vi "Vision Processing.vi"(4 "error in (no error)":errorcluster, 7 "Image Size":T3=enum."320x240") -> (2 "Target Y":dbl, 3 "Target  X":dbl)   [LabVIEW 2015]
uses:
  <vilib>/Rock Robotics/WPI/Camera/WPI_CameraImageSize.ctl
  <vilib>/Rock Robotics/WPI/Camera/WPI_CameraWhite Balance Values.ctl
  <vilib>/Rock Robotics/WPI/Camera/WPI_CameraExposure Values.ctl
  <vilib>/Rock Robotics/WPI/Camera/WPI_CameraFrameRate.ctl
  Vision Support Code/Camera Types.ctl
  Robot Global Data.vi
  <vilib>/vision/NI_Vision_Development_Module.lvlib
panel:
  out "Highest Avg Score":dbl
  in  "Min Score Threshold":i32=75
  out "Detected Targets":T1(array[cluster]) {"Normalized Rect"."Numeric 5" format="%#_2g"; "Normalized Rect"."Numeric 3" format="%#_2g"; "Normalized Rect"."Numeric 2" format="%#_2g"; "Normalized Rect"."Numeric" format="%#_2g"}
  out "Sorted Particle Scores":T2(array[cluster]) {"Moment Factor" format="%#_3g"; "Aspect Ratio" format="%#_3g"; "Area to CH" format="%#_3g"; "X" format="%#_3g"; "Y" format="%#_3g"}
  in  "Display Original":bool=TRUE
  in  "Display Mask":bool=TRUE
  out "fps":dbl
  in  "Emphasize Limit Tests":bool=TRUE
  in  "Aspect Fudge Factor":dbl=1.0
  in  "Score Threshold":dbl=75.0
  out "ms to process":u32
  out "Qualified Particles":i32
  in  "LED Color":T4={"Hue"={111.0, 149.0}, "Sat"={35.0, 255.0}, "Val"={93.0, 255.0}} {"Hue" scale=0.0..255.0 scale format="%#_3g"}
  out "Masked":T5(plugin-control)
  out "Original Image":T5(plugin-control)
  # "NOTE:\nFor best results, lower the camera\nexposure."
  # "This is only the initial camera size.\nOther camera setup is done\non the diagram. Notice it is set\nonce before the loop but can be\nupdated within the loop if needed."
  # "Instructions:\nUse LED Color to threshold and build particles. Adjust calibration if needed.\nDisplays are very useful for debugging, but will slow down execution, so you\nmay want to disable once working.\nAnnotations show the rectangle and the scores from top to bottom.\nChange camera setting on diagram."
  # "x"
  # "y"
  # "Density Profile"
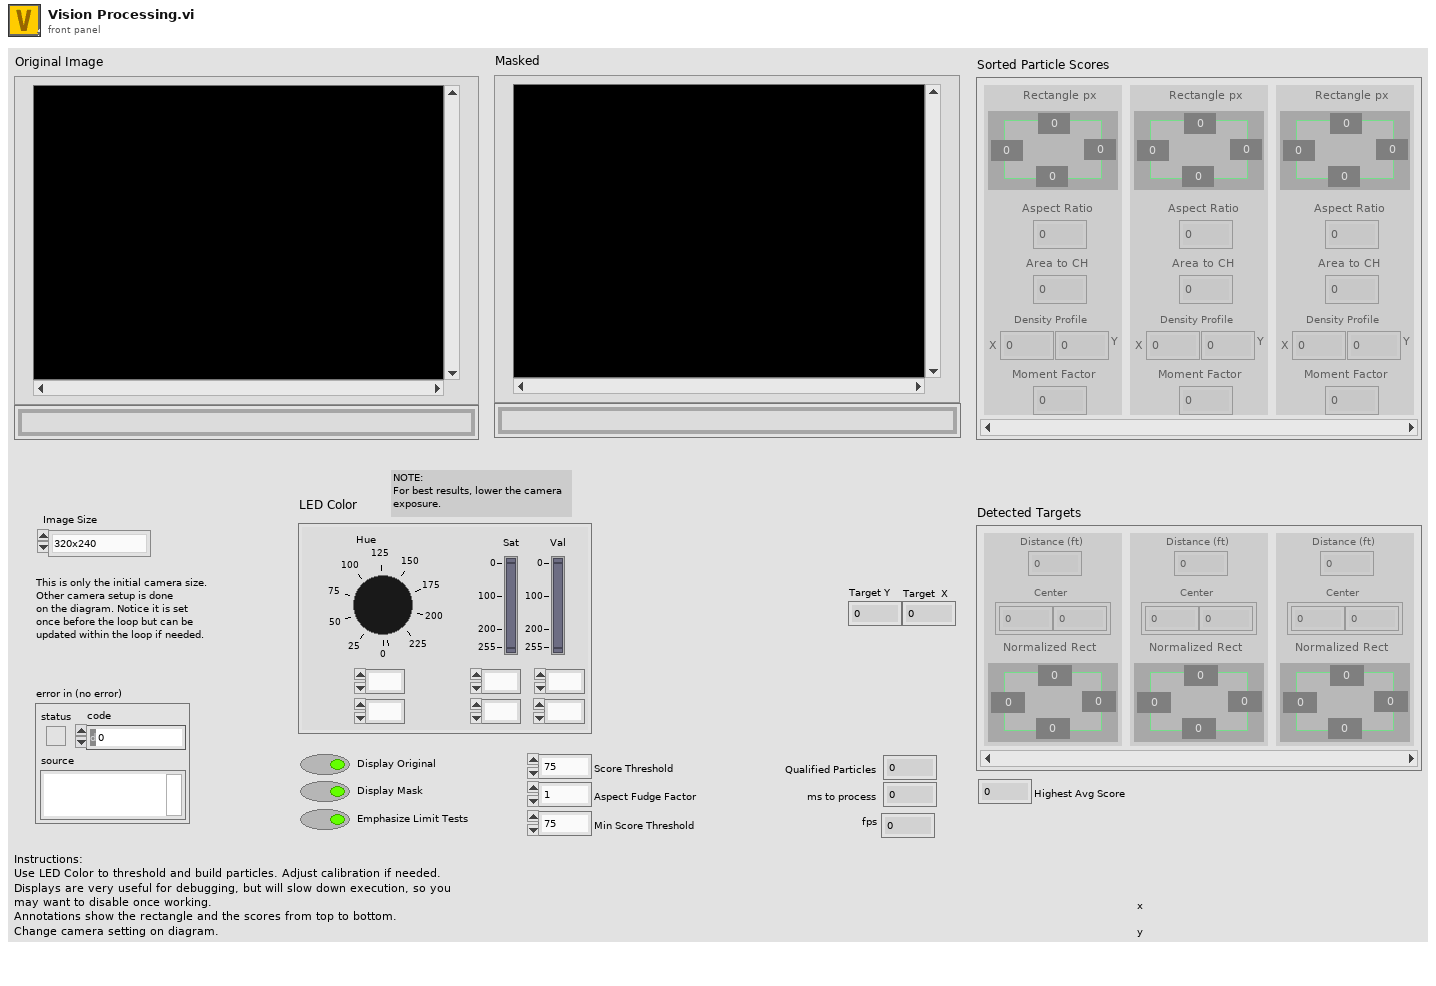
[diagram p1: front panel]
types:
  T1 = cluster{"Distance (ft)":dbl, "Center":cluster{dbl, dbl}, "Normalized Rect":cluster{"Numeric":dbl, "Numeric 2":dbl, "Numeric 3":dbl, "Numeric 5":dbl}}[]
  T2 = cluster{"Rectangle px":cluster{"Numeric":dbl, "Numeric 2":dbl, "Numeric 3":dbl, "Numeric 5":dbl}, "Aspect Ratio":dbl, "Area to CH":dbl, "X":dbl, "Y":dbl, "Moment Factor":dbl}[]
  T3 = typedef "WPI_CameraImageSize.ctl" = enum16{"640x480", "320x240", "160x120", "Custom"}
  T4 = cluster{"Hue":cluster{dbl, dbl}, "Sat":cluster{dbl, dbl}, "Val":cluster{dbl, dbl}}
  T5 = typedef "IMAQ Image.ctl" = refnum<image>
  T6 = typedef "WPI_CameraFrameRate.ctl" = u32
  T7 = typedef "WPI_CameraExposure Values.ctl" = enum16{"Auto", "Flicker-free 50 Hz", "Flicker-free 60 Hz", "Hold current", "Custom"}
  T8 = typedef "WPI_CameraWhite Balance Values.ctl" = enum16{"Auto", "Fixed indoor", "Fixed outdoor 1", "Fixed outdoor 2", "Fixed fluorescent 1", "Fixed fluorescent 2", "Hold current", "Custom"}
  T9 = typedef "Particle Parameters" = i32
  T10 = typedef "Image Type" = u32
  T11 = typedef "WPI_CameraDevRef.ctl" = cluster{"Camera Address":string, "CameraStatus":errorcluster}
  T12 = typedef "Camera Types.ctl" = enum16{"206", "1011", "1013", "MS HD3000 square", "MS HD3000 640x480"}
  T13 = cluster{"Bounding box":cluster{"left":dbl, "top":dbl, "right":dbl, "bottom":dbl}, "Aspect Ratio":dbl, "Area to CH":dbl, "X Mask":dbl, "Y Mask":dbl, "Moment":dbl}[]
  T14 = cluster{"Rectangle":cluster{"Numeric":dbl, "Numeric 2":dbl, "Numeric 3":dbl, "Numeric 5":dbl}, "L":dbl, "Area to CH":dbl, "X":dbl, "Y":dbl, "Moment Factor":dbl}[]
  T15 = cluster{"Distance (ft)":dbl, "Center":cluster{dbl, dbl}, "Normalized Rect":cluster{"Numeric":dbl, "Numeric 2":dbl, "Numeric 3":dbl, "Numeric 5":dbl}}
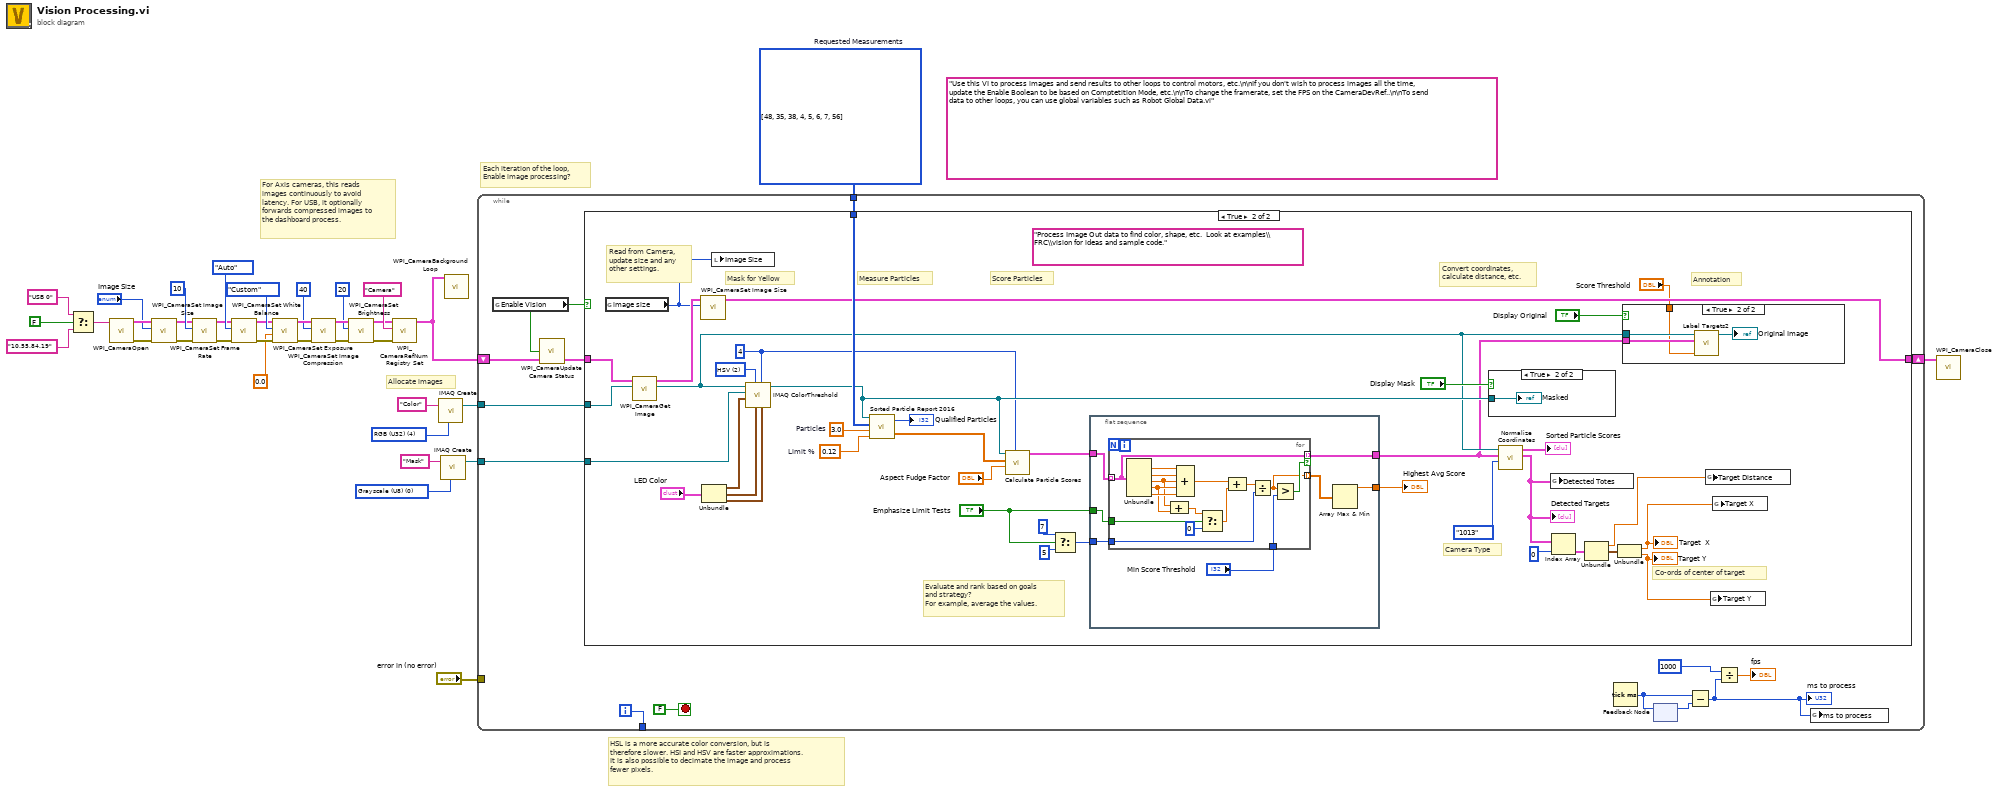
[diagram p0: block diagram]
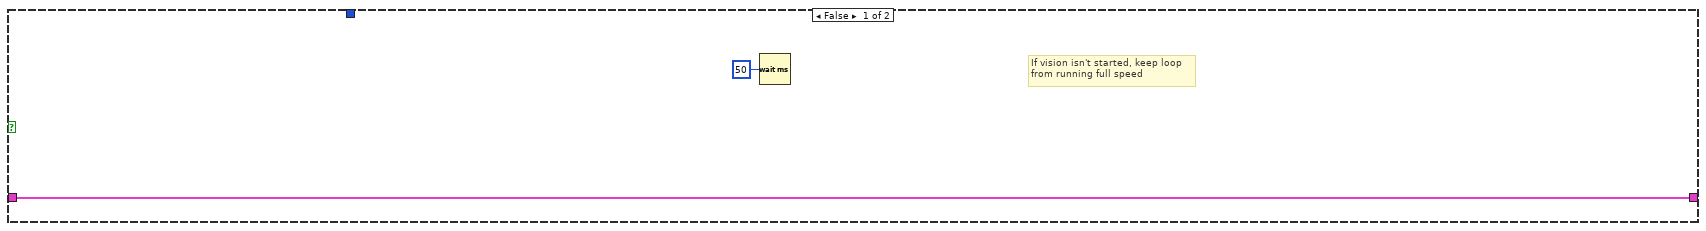
[diagram p2: hidden frame]
diagram:
  (unwired) "Use this VI to process images and send results to other loops to control motors, etc.\n\nIf you don't wish to process images all the time, update the Enable Boolean to be based on Comptetition Mode, etc.\n\nTo change the framerate, set the FPS on the CameraDevRef..\n\nTo send data to other loops, you can use global variables such as Robot Global Data.vi"
  w30 = T9[] [48, 35, 38, 4, 5, 6, 7, 56] items=["Center of Mass X", "Center of Mass Y", "First Pixel X", "First Pixel Y", "Bounding Rect Left", "Bounding Rect Top", "Bounding Rect Right", "Bounding Rect Bottom", "Max Feret Diameter Start X", "Max Feret Diameter Start Y", "Max Feret Diameter End X", "Max Feret Diameter End Y", "Max Horiz. Segment Length Left", "Max Horiz. Segment Length Right", "Max Horiz. Segment Length Row", "-", "Bounding Rect Width", "Bounding Rect Height", "Bounding Rect Diagonal", "Perimeter", "Convex Hull Perimeter", "Holes' Perimeter", "Max Feret Diameter", "Equivalent Ellipse Major Axis", "Equivalent Ellipse Minor Axis", "Equivalent Ellipse Minor Axis (Feret)", "Equivalent Rect Long Side", "Equivalent Rect Short Side", "Equivalent Rect Diagonal", "Equivalent Rect Short Side (Feret)", "Average Horiz. Segment Length", "Average Vert. Segment Length", "Hydraulic Radius", "Waddel Disk Diameter", "-", "Area", "Holes' Area", "Particle & Holes' Area", "Convex Hull Area", "Image Area", "-", "Number of Holes", "Number of Horiz. Segments", "Number of Vert. Segments", "-", "Orientation", "Max Feret Diameter Orientation", "-", "% Area/Image Area", "% Area/(Particle & Holes' Area)", "Ratio of Equivalent Ellipse Axes", "Ratio of Equivalent Rect Sides", "-", "Elongation Factor", "Compactness Factor", "Heywood Circularity Factor", "Type Factor", "-", "Sum X", "Sum Y", "Sum XX", "Sum XY", "Sum YY", "Sum XXX", "Sum XXY", "Sum XYY", "Sum YYY", "-", "Moment of Inertia XX", "Moment of Inertia XY", "Moment of Inertia YY", "Moment of Inertia XXX", "Moment of Inertia XXY", "Moment of Inertia XYY", "Moment of Inertia YYY", "Norm. Moment of Inertia XX", "Norm. Moment of Inertia XY", "Norm. Moment of Inertia YY", "Norm. Moment of Inertia XXX", "Norm. Moment of Inertia XXY", "Norm. Moment of Inertia XYY", "Norm. Moment of Inertia YYY", "Hu Moment 1", "Hu Moment 2", "Hu Moment 3", "Hu Moment 4", "Hu Moment 5", "Hu Moment 6", "Hu Moment 7"]  # Requested Measurements
  w33 = T10 0 items=["Grayscale (U8)", "Grayscale (I16)", "Grayscale (SGL)", "Complex (CSG)", "RGB (U32)", "HSL (U32)", "RGB (U64)", "Grayscale (U16)"] ("Image Type")
  w35 = T10 4 items=["Grayscale (U8)", "Grayscale (I16)", "Grayscale (SGL)", "Complex (CSG)", "RGB (U32)", "HSL (U32)", "RGB (U64)", "Grayscale (U16)"] ("Image Type")
  # "Each iteration of the loop,\nEnable image processing?"
  # "HSL is a more accurate color conversion, but is\ntherefore slower. HSI and HSV are faster approximations.\nIt is also possible to decimate the image and process\nfewer pixels."
  # "For Axis cameras, this reads\nimages continuously to avoid\nlatency. For USB, it optionally\nforwards compressed images to\nthe dashboard process."
  # "Allocate images"
  n1 = Select(t="USB 0" ("format string"), s=FALSE ("dot notation? (F)"), f="10.55.84.19" ("format string")) -> (s? t:f=w29:string)
  n2 = call <vilib>:"WPI_CameraOpen.vi"("Camera Address"=w29) -> ("error out"=w17:errorcluster, "CameraDevRef"=w16:T11)  [unwired: 1 in, 8 out]
  n3 = call <vilib>:"WPI_CameraSet Image Size.vi"("error in (no error)"=w17, "Image Size"="Image Size", "CameraDevRef"=w16) -> ("error out"=w18:errorcluster, "CameraDevRef Out"=w15:T11)  [unwired: 1 in, 6 out]
  n4 = call <vilib>:"WPI_CameraSet Frame Rate.vi"("error in (no error)"=w18, "Frame Rate (fps)"=T6 10, "CameraDevRef"=w15) -> ("error out"=w19:errorcluster, "CameraDevRef Out"=w13:T11)  [unwired: 7 out]
  n5 = call <vilib>:"WPI_CameraSet White Balance.vi"("error in (no error)"=w19, "White Balance"=WPI_CameraWhite_Balance_Values."Auto", "CameraDevRef"=w13) -> ("error out"=w20:errorcluster, "CameraDevRef Out"=w14:T11)  [unwired: 1 in, 6 out]
  n6 = call <vilib>:"WPI_CameraSet Exposure.vi"("error in (no error)"=w20, "Exposure (%)"=0.0, "Exposure"=WPI_CameraExposure_Values."Custom", "CameraDevRef"=w14) -> ("error out"=w21:errorcluster, "CameraDevRef Out"=w11:T11)  [unwired: 6 out]
  n7 = call <vilib>:"WPI_CameraSet Image Compression.vi"("error in (no error)"=w21, "Compression"=40, "CameraDevRef"=w11) -> ("error out"=w22:errorcluster, "CameraDevRef Out"=w12:T11)  [unwired: 7 out]
  n8 = call <vilib>:"WPI_CameraSet Brightness.vi"("error in (no error)"=w22, "Brightness"=20, "CameraDevRef"=w12) -> ("error out"=w23:errorcluster, "CameraDevRef Out"=w2:T11)  [unwired: 7 out]
  n9 = call <vilib>:"WPI_CameraRefNum Registry Set.vi"("error in (no error)"=w23, "refnum name"="Camera", "CameraDevRef"=w2) -> ("CameraDevRef"=w7:T11)  [unwired: 1 in, 7 out]
  n10 = call "IMAQ Create"("Image Name"="Color", "Image Type"=w35) -> ("New Image"=w34:T5)  [unwired: 2 in, 2 out]
  n11 = call "IMAQ Create"("Image Name"="Mask", "Image Type"=w33) -> ("New Image"=w31:T5)  [unwired: 2 in, 2 out]
  n12 = call <vilib>:"WPI_CameraBackground Loop.vi"("CameraDevRef"=w7) -> ()  [unwired: 11 in]
  n13 = while {
    tunnel: w34 -> [w45]
    tunnel: w31 -> [w49]
    tunnel: w30 -> [w48]
    tunnel: "error in (no error)" -> [_]
    tunnel: [w44] -> _
    shift-right: [w40] -> w3
    shift-left: w7 -> [w42]
    i -> [w44]
    stop <- FALSE stop-if-true
    n14 = global read "Robot Global Data.vi" "Enable Vision"() -> (w43:bool)
    n15 = call <vilib>:"WPI_CameraUpdate Camera Status.vi"("CameraDevRef In"=w42, "Enable Vision"=w43) -> ("CameraDevRef Out"=w41:T11)  [unwired: 3 in]
    n16 = case shown="True" w43 {
      tunnel: w49 -> [_ w91]
      tunnel: w48 -> [_ w86]
      tunnel: w41 -> [w51 w82]
      tunnel: w45 -> [_ w81]
      tunnel: [w51 w79] -> w40
      frame False {
        # "If vision isn't started, keep loop\nfrom running full speed"
        n17 = Wait (ms)(milliseconds to wait=u32 50) -> ()  [unwired: 1 out]
      }
      frame True {
        w63 = 4 ("Replace Value")
        w76 = u16 2 items=["RGB", "HSL", "HSV", "HSI"] ("Color Mode")
        (unwired) "Process Image Out data to find color, shape, etc.  Look at examples\\FRC\\vision for ideas and sample code."
        w83 = 0.12  # Limit %
        w85 = 3.0  # Particles
        # "Co-ords of center of target"
        # "Camera Type"
        # "Evaluate and rank based on goals\nand strategy?\nFor example, average the values."
        # "Read from Camera,\nupdate size and any\nother settings."
        # "Measure Particles"
        # "Convert coordinates,\ncalculate distance, etc."
        # "Annotation"
        # "Score Particles"
        # "Mask for Yellow"
        n18 = global read "Robot Global Data.vi" "image size"() -> (w62:T3)
        n19 = call <vilib>:"WPI_CameraGet Image.vi"("Image"=w81, "CameraDevRef"=w82) -> ("Image Out"=w66:T5, "CameraDevRef Out"=w80:T11)  [unwired: 7 in, 1 out]
        n20 = call <vilib>:"WPI_CameraSet Image Size.vi"("Image Size"=w62, "CameraDevRef"=w80) -> ("CameraDevRef Out"=w79:T11)  [unwired: 2 in, 7 out]
        n21 = Unbundle("LED Color") -> ("Hue"=w90:cluster{dbl, dbl}, "Sat"=w89:cluster{dbl, dbl}, "Val"=w88:cluster{dbl, dbl})
        n22 = local write "Image Size"(w62) -> ()
        n23 = call "IMAQ ColorThreshold"("Blue or Luma or Val or Inten Range"=w88, "Replace Value"=w63, "Green or Sat Range"=w89, "Color Mode"=w76, "Red or Hue Range"=w90, "Image Dst"=w91, "Image Src"=w66) -> ("Image Dst Out"=w75:T5)  [unwired: 3 in, 1 out]
        n24 = call "Sorted Particle Report 2016.vi"("Min Area Size %"=w83, "Particle Count Limit"=w85, "Pixel Measurements"=w86, "Image in"=w75) -> ("Sorted Data"=w74:dbl[][], "Particles"=→"Qualified Particles":i32)
        n25 = call "Calculate Particle Scores.vi"("Pixel Value"=w63, "Aspect Fudge Factor"="Aspect Fudge Factor", "Sorted Data"=w74, "Image in"=w75) -> ("Scores"=w72:T13)  [unwired: 7 in]
        n26 = Select(t=7, s="Emphasize Limit Tests", f=5) -> (s? t:f=w69:i32)
        n27 = flat-sequence {
          tunnel: w72 -> [w102]
          tunnel: w69 -> [w100]
          tunnel: [w103] -> w68
          tunnel: [w97] -> w65
          tunnel: "Emphasize Limit Tests" -> [w101]
          frame #0 {
            n28 = for {
              tunnel: w102 -> [w117] mode=indexing
              tunnel: [w117] -> w97 mode=indexing if=w116
              tunnel: [w115] -> w98 mode=indexing
              tunnel: w100 -> [w114]
              tunnel: "Min Score Threshold" -> [w113]
              tunnel: w101 -> [w106]
              n29 = Unbundle(w117) -> ("Aspect Ratio"=w119:dbl, "Area to CH"=w118:dbl, "X Mask"=w108:dbl, "Y Mask"=w109:dbl, "Moment"=w110:dbl)  [unwired: 1 out]
              n30 = Compound Arithmetic op=ADD(w108, w109) -> (w107:dbl)
              n31 = Compound Arithmetic op=ADD(w119, w118, w108, w109, w110) -> (w112:dbl)
              n32 = Select(t=w107, s=w106, f=0) -> (s? t:f=w105:dbl)
              n33 = Compound Arithmetic op=ADD(w112, w105) -> (w111:dbl)
              n34 = Divide(x=w111, y=w114) -> (x/y=w115:dbl)
              n35 = Greater?(x=w115, y=w113) -> (0:w116:bool)
            }
            n36 = Array Max & Min(array=w98) -> (max value=w103:dbl)  [unwired: 3 out]
          }
        }
        n37 = case shown="True" "Display Mask" {
          tunnel: w75 -> [_ w96]
          frame False {
          }
          frame True {
            "Masked" <- w96
          }
        }
        n38 = call "Normalize Coordinates.vi"("Camera Type"=Camera_Types."1013", "Targets"=w65, "Image in"=w66) -> ("Found Targets"=w59:T1, "Sorted Scores"=→"Sorted Particle Scores":T14)  [unwired: 7 in]
        "Detected Targets" <- w59
        n39 = global write "Robot Global Data.vi" "Detected Totes"(w59) -> ()
        n40 = Index Array(array=w59, index=0) -> (element=w57:T15)
        n41 = Unbundle(w57) -> ("Distance (ft)"=w53:dbl, "Center"=w56:cluster{dbl, dbl})  [unwired: 1 out]
        n42 = Unbundle(w56) -> (w55:dbl, w54:dbl)
        "Target  X" <- w55
        "Target Y" <- w54
        n43 = case shown="True" "Display Original" {
          tunnel: w66 -> [_ w95]
          tunnel: w65 -> [_ w93]
          tunnel: "Score Threshold" -> [_ w92]
          frame False {
          }
          frame True {
            n44 = call "Label Targets2.vi"("Score Threshold"=w92, "Targets"=w93, "Image in"=w95) -> ("Image out"=→"Original Image":T5)  [unwired: 8 in]
          }
        }
        n45 = global write "Robot Global Data.vi" "Target Distance"(w53) -> ()
        n46 = global write "Robot Global Data.vi" "Target Y"(w54) -> ()
        n47 = global write "Robot Global Data.vi" "Target X"(w55) -> ()
        "Highest Avg Score" <- w68
      }
    }
    n48 = Tick Count (ms)() -> (millisecond timer value=w46:u32)
    n49 = feedback-in #1(w46) -> ()
    n50 = feedback #1() -> (w47:u32)  [unwired: 1 in]
    n51 = Subtract(x=w46, y=w47) -> (x-y=w39:u32)
    "ms to process" <- w39
    n52 = Divide(x=1000 ("Brightness"), y=w39) -> (x/y=→"fps":dbl)
    n53 = global write "Robot Global Data.vi" "ms to process"(w39) -> ()
  }
  n54 = call <vilib>:"WPI_CameraClose.vi"("CameraDevRef"=w3) -> ()  [unwired: 1 in, 10 out]
